vi "PNEU_Write_Close.vi"(0 "Pneu":T1) -> ()   [LabVIEW 2015]
uses:
  Periodic Task/Ref_Num/Pneu_Type_Def.ctl
  <vilib>/Rock Robotics/WPI/Solenoid/WPI_SolenoidDevRef.ctl
  <vilib>/Rock Robotics/WPI/Solenoid/WPI_SolenoidChannel.ctl
  <vilib>/Rock Robotics/WPI/Compressor/WPI_CompressorDevRef.ctl
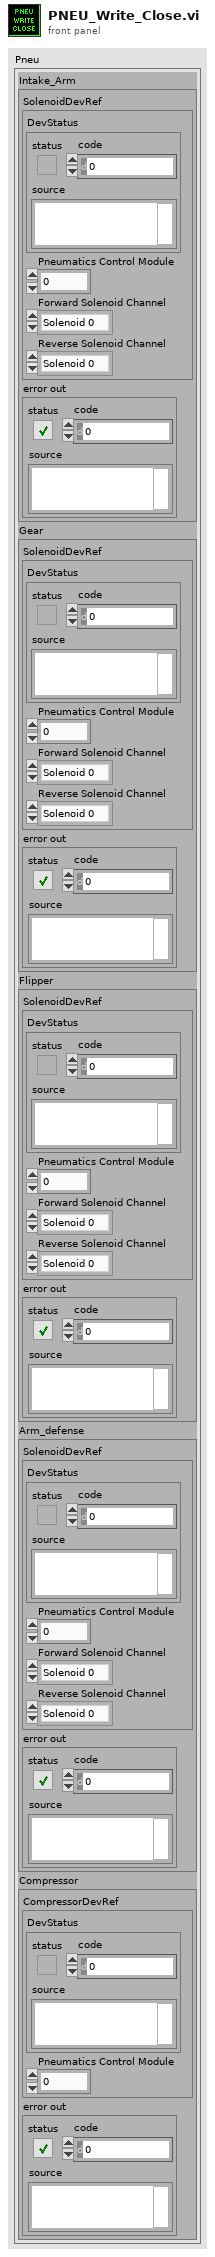
[diagram p1: front panel]
types:
  T1 = typedef "Pneu_Type_Def.ctl" = cluster{"Intake_Arm":cluster{"SolenoidDevRef":T2, "error out":errorcluster}, "Gear":cluster{"SolenoidDevRef":T2, "error out":errorcluster}, "Flipper":cluster{"SolenoidDevRef":T2, "error out":errorcluster}, "Arm_defense":cluster{"SolenoidDevRef":T2, "error out":errorcluster}, "Compressor":cluster{"CompressorDevRef":T4, "error out":errorcluster}}
  T2 = typedef "WPI_SolenoidDevRef.ctl" = cluster{"DevStatus":errorcluster, "Pneumatics Control Module":u8, "Forward Solenoid Channel":T3, "Reverse Solenoid Channel":T3}
  T3 = typedef "WPI_SolenoidChannel.ctl" = enum8{"Solenoid 0", "Solenoid 1", "Solenoid 2", "Solenoid 3", "Solenoid 4", "Solenoid 5", "Solenoid 6", "Solenoid 7", "Invalid"}
  T4 = typedef "WPI_CompressorDevRef.ctl" = cluster{"DevStatus":errorcluster, "Pneumatics Control Module":u8}
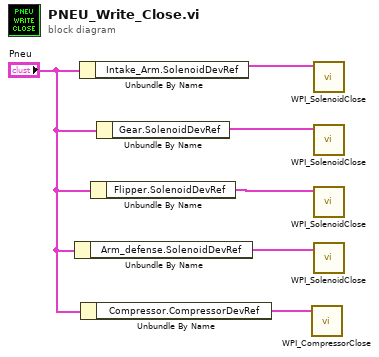
[diagram p0: block diagram]
diagram:
  n1 = Unbundle By Name("Pneu") -> ("Arm_defense.SolenoidDevRef"=w3:T2)
  n2 = Unbundle By Name("Pneu") -> ("Intake_Arm.SolenoidDevRef"=w6:T2)
  n3 = Unbundle By Name("Pneu") -> ("Compressor.CompressorDevRef"=w1:T4)
  n4 = Unbundle By Name("Pneu") -> ("Flipper.SolenoidDevRef"=w4:T2)
  n5 = Unbundle By Name("Pneu") -> ("Gear.SolenoidDevRef"=w5:T2)
  n6 = call <vilib>:"WPI_CompressorClose.vi"("CompressorDevRef"=w1) -> ()  [unwired: 10 in, 1 out]
  n7 = call <vilib>:"WPI_SolenoidClose.vi"("SolenoidDevRef"=w6) -> ()  [unwired: 10 in, 1 out]
  n8 = call <vilib>:"WPI_SolenoidClose.vi"("SolenoidDevRef"=w5) -> ()  [unwired: 10 in, 1 out]
  n9 = call <vilib>:"WPI_SolenoidClose.vi"("SolenoidDevRef"=w4) -> ()  [unwired: 10 in, 1 out]
  n10 = call <vilib>:"WPI_SolenoidClose.vi"("SolenoidDevRef"=w3) -> ()  [unwired: 10 in, 1 out]
